vi "TagContainer-ReadAsVariant.vi"(8 "error in (no error)":errorcluster, 10 "name":string, 11 "TagContainer":T1) -> (0 "error out":errorcluster, 1 "found":bool, 2 "Value":variant, 3 "TagContainer(dup)":T1, 4 "Time Stamp":timestamp, 5 "Raw name":string)   [LabVIEW 2017, in "TagContainer.lvlib"]
uses:
  TagContainer.lvlib
  Typedef/TagContainer.ctl
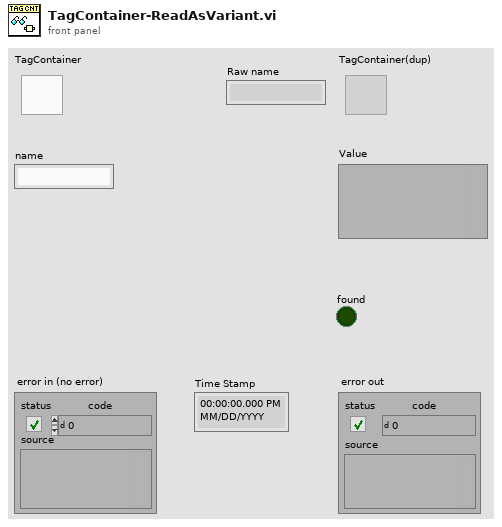
[diagram p1: front panel]
types:
  T1 = typedef "TagContainer.lvlib/TagContainer.ctl" = refnum<k1>
  T2 = typedef "tagcontainer-data.ctl" = cluster{"tag-map":variant, "timestamp-map":variant}
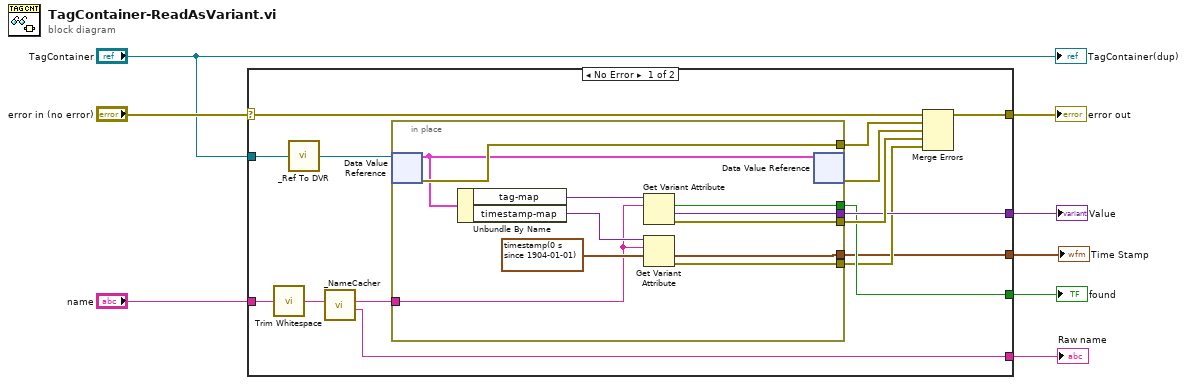
[diagram p0: block diagram]
diagram:
  n1 = case shown="No Error" "error in (no error)" {
    selector: "error in (no error)" -> [w21 w35]
    tunnel: [w22 w35] -> w7
    tunnel: "name" -> [w18 _]
    tunnel: "TagContainer" -> [w17 _]
    tunnel: [w16 _] -> w5
    tunnel: [w15 _] -> w4
    tunnel: [w12 _] -> w2
    tunnel: [w10 _] -> w1
    frame No Error {
      n2 = call <vilib>:"Trim Whitespace.vi"("string"=w18) -> ("trimmed string"=w9:string)  [unwired: 1 in]
      n3 = call "_Ref To DVR.vi"("TagContainer"=w17) -> ("DVR"=w14:refnum<data-value>)
      n4 = call "_NameCacher.vi"("key"=w9) -> ("Raw name"=w10:string, "Key in lower case"=w11:string)  [unwired: 8 in, 1 out]
      n5 = in-place "In Place Element Structure" {
        in-place-border: w11 -> [w26]
        in-place-border: [w33] -> w19
        in-place-border: [w34] -> w23
        in-place-border: [w32] -> w16
        in-place-border: [w31] -> w15
        in-place-border: [w25] -> w13
        in-place-border: [w24] -> w12
        n6 = in-place-dvr #1(w14) -> (w30:T2, w33:errorcluster)
        n7 = Unbundle By Name(w30) -> ("tag-map"=w29:variant, "timestamp-map"=w28:variant)
        n8 = Get Variant Attribute(Variant=w29, name=w26) -> (found=w31:bool, value=w32:variant, error out=w34:errorcluster)  [unwired: 2 in, 1 out]
        n9 = Get Variant Attribute(Variant=w28, name=w26, default value (empty Variant)=timestamp(0 s since 1904-01-01) ("Time Stamp")) -> (value=w24:timestamp, error out=w25:errorcluster)  [unwired: 1 in, 2 out]
        n10 = in-place-dvr #1(w30) -> (w20:errorcluster)  [unwired: 1 out]
      }
      n11 = Merge Errors(w21, w19, w20, w23, w13) -> (w22:errorcluster)
    }
    frame Error {
    }
  }
  "error out" <- w7
  "Value" <- w5
  "found" <- w4
  "Time Stamp" <- w2
  "Raw name" <- w1
  "TagContainer(dup)" <- "TagContainer"
